vi "Add State (to Dictionaries).vi"(8 "error in":errorcluster, 10 "state and connections":T1, 11 "routing channel in":T3 format="%.0x") -> (0 "error out":errorcluster, 3 "routing channel out":T3=18446744073709551615 format="%.0x")   [LabVIEW 2020, in "Routing and Faulting Scripting.lvlib"]
uses:
  Routing and Faulting Scripting.lvlib
  <vilib>/NI VeriStand/Custom Device API/Custom Device Item Ref.ctl
  Shared/Routing State.ctl
  Shared/Connection.ctl
  NationalInstruments.VeriStand.SystemDefinitionAPI
  Constants/Scripting Constants.vi
  Utility/Connection to String.vi
  <vilib>/NI VeriStand/Custom Device API/Custom Device API.lvlib
  Shared/Routing and Faulting Shared.lvlib
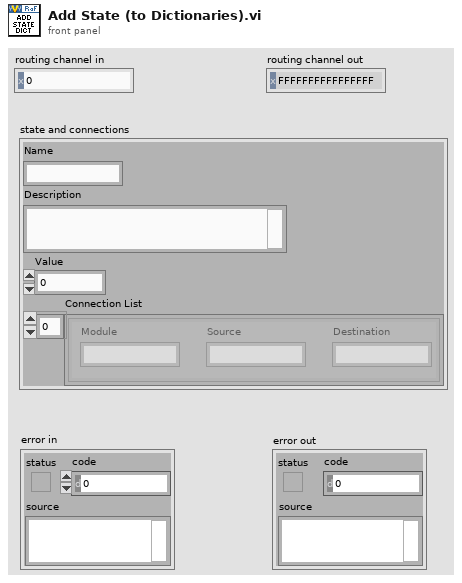
[diagram p1: front panel]
types:
  T1 = typedef "Routing and Faulting Shared.lvlib/Routing State.ctl" = cluster{"Name":string, "Description":string, "Value":i32, "Connection List":T2[]}
  T2 = typedef "Routing and Faulting Shared.lvlib/Connection.ctl" = cluster{"Module":string, "Source":string, "Destination":string}
  T3 = typedef "Custom Device API.lvlib/Custom Device Item Ref.ctl" = u64
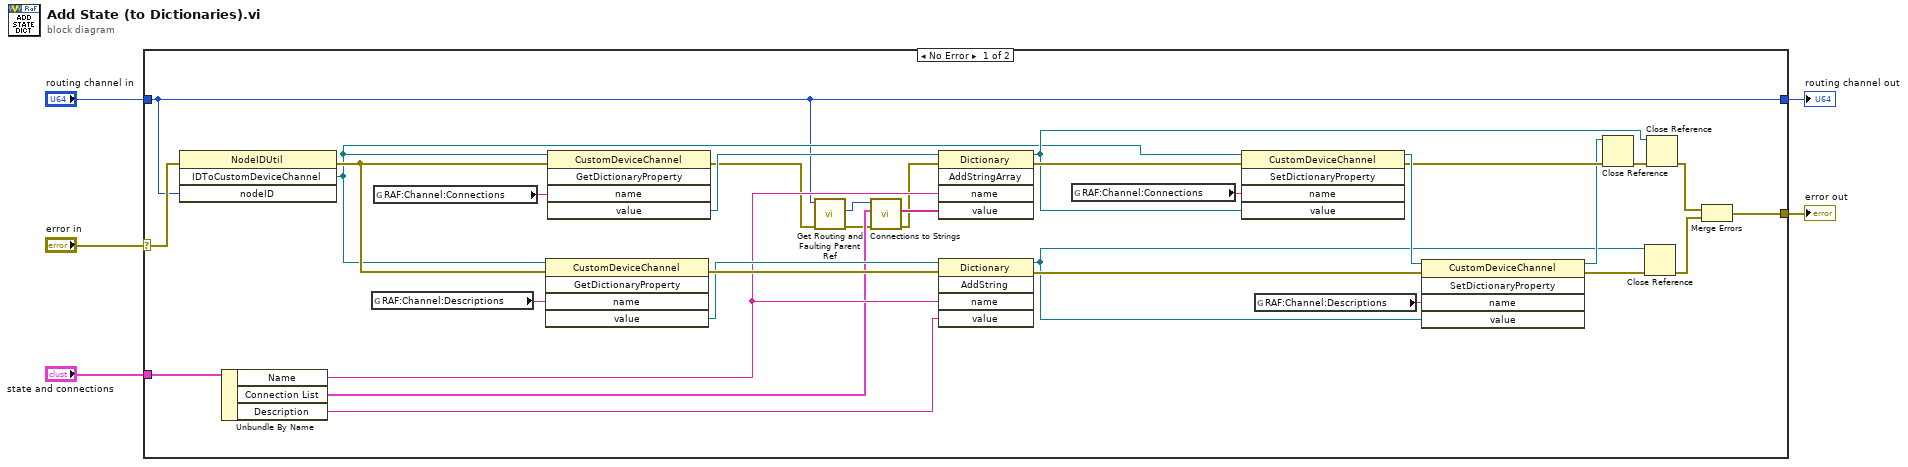
[diagram p0: block diagram]
diagram:
  n1 = case shown="No Error" "error in" {
    selector: "error in" -> [w36 w39]
    tunnel: [w17 w39] -> w4
    tunnel: "routing channel in" -> [w7 w38]
    tunnel: [w7 w38] -> w2
    tunnel: "state and connections" -> [w15 _]
    frame No Error {
      n2 = invoke class="NodeIDUtil" method="IDToCustomDeviceChannel"(error in=w36, "nodeID"=w7) -> (error out=w28:errorcluster, "IDToCustomDeviceChannel"=w25:refnum<k24>)  [unwired: 2 in, 2 out]
      n3 = Unbundle By Name(w15) -> ("Name"=w14:string, "Connection List"=w12:T2[], "Description"=w13:string)
      n4 = global read "Scripting Constants.vi" "RAF:Channel:Descriptions"() -> (w29:string)
      n5 = global read "Scripting Constants.vi" "RAF:Channel:Connections"() -> (w34:string)
      n6 = invoke class="CustomDeviceChannel" method="GetDictionaryProperty"(reference=w25, error in=w28, "name"=w29) -> (error out=w27:errorcluster, "value"=w26:refnum<k24>)  [unwired: 2 in, 3 out]
      n7 = invoke class="CustomDeviceChannel" method="GetDictionaryProperty"(reference=w25, error in=w28, "name"=w34) -> (error out=w9:errorcluster, "value"=w16:refnum<k24>)  [unwired: 2 in, 3 out]
      n8 = call "Get Routing and Faulting Parent Ref.vi"("error in"=w9, "routing and faulting child in"=w7) -> ("error out"=w8:errorcluster, "routing and faulting"=w6:T3)  [unwired: 7 in, 1 out]
      n9 = call "Connections to Strings.vi"("error in"=w8, "connection list"=w12, "routing and faulting in"=w6) -> ("error out"=w10:errorcluster, "connection strings"=w11:string[])  [unwired: 6 in, 1 out]
      n10 = invoke class="Dictionary" method="AddStringArray"(reference=w16, error in=w10, "name"=w14, "value"=w11) -> (reference out=w32:refnum<k24>, error out=w35:errorcluster)  [unwired: 1 in, 3 out]
      n11 = invoke class="Dictionary" method="AddString"(reference=w26, error in=w27, "name"=w14, "value"=w13) -> (reference out=w21:refnum<k24>, error out=w30:errorcluster)  [unwired: 1 in, 3 out]
      n12 = global read "Scripting Constants.vi" "RAF:Channel:Connections"() -> (w33:string)
      n13 = invoke class="CustomDeviceChannel" method="SetDictionaryProperty"(reference=w25, error in=w35, "name"=w33, "value"=w32) -> (reference out=w24:refnum<k24>, error out=w23:errorcluster)  [unwired: 1 in, 3 out]
      n14 = global read "Scripting Constants.vi" "RAF:Channel:Descriptions"() -> (w31:string)
      n15 = invoke class="CustomDeviceChannel" method="SetDictionaryProperty"(reference=w24, error in=w30, "name"=w31, "value"=w21) -> (reference out=w22:refnum<k24>, error out=w20:errorcluster)  [unwired: 1 in, 3 out]
      n16 = Close Reference(reference=w22, error in (no error)=w23) -> (error out=w37:errorcluster)
      n17 = Close Reference(reference=w21, error in (no error)=w20) -> (error out=w18:errorcluster)
      n18 = Close Reference(reference=w32, error in (no error)=w37) -> (error out=w19:errorcluster)
      n19 = Merge Errors(w19, w18) -> (w17:errorcluster)
    }
    frame Error {
    }
  }
  "routing channel out" <- w2
  "error out" <- w4
